vi "open default configuration.vi"(4 "error in (not an error)":errorcluster, 7 "Sensor Array":T1) -> (0 "error out":errorcluster, 3 "Sensor Array out":T1)   [LabVIEW 2012]
uses:
  DAQ configuration/Sensor array.ctl
  DAQ configuration/channel identifier.ctl
  DAC project/Calibration and Function folders.ctl
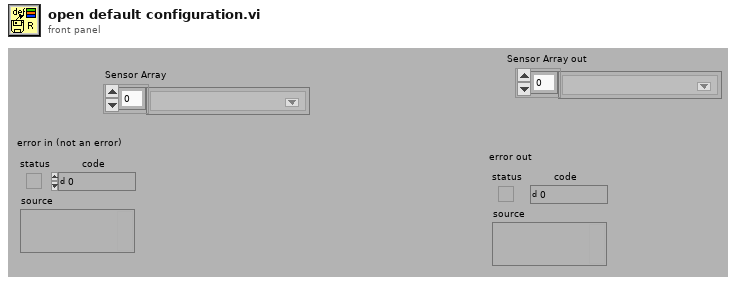
[diagram p1: front panel]
types:
  T1 = typedef "Sensor array.ctl" = T2[]
  T2 = typedef "channel identifier.ctl" = u16
  T3 = typedef "Calibration and Function folders.ctl" = enum16{"Sensors", "Functions", "Config File", "UserAppFolder"}
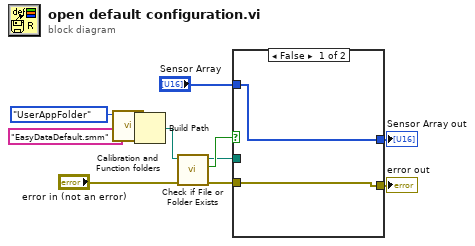
[diagram p0: block diagram]
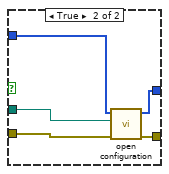
[diagram p2: hidden frame]
diagram:
  n1 = call "Calibration and Function folders.vi"("Folder"=Calibration_and_Function_folders."UserAppFolder") -> ("Selected Folder"=w1:path)  [unwired: 10 in]
  n2 = Build Path(base path=w1, name or relative path="EasyDataDefault.smm") -> (appended path=w10:path)
  n3 = call <vilib>:"Check if File or Folder Exists.vi"("error in (no error)"="error in (not an error)", "path"=w10) -> ("error out"=w8:errorcluster, "file or folder exists?"=w5:bool, "dup path"=w4:path)  [unwired: 7 in]
  n4 = case shown="False" w5 {
    tunnel: w8 -> [w13 w18]
    tunnel: [w12 w17] -> w7
    tunnel: [w13 w16] -> w6
    tunnel: w4 -> [_ w15]
    tunnel: "Sensor Array" -> [w12 w14]
    frame False {
    }
    frame True {
      n5 = call "open configuration.vi"("error in"=w18, "file path"=w15, "Sensor Array"=w14) -> ("error out"=w16:errorcluster, "Sensor Array out"=w17:T1)  [unwired: 3 in]
    }
  }
  "error out" <- w6
  "Sensor Array out" <- w7
